vi "UI Initialize.vi"(8 "error in (no error)":errorcluster, 11 "UI ActorTop in":refnum<class "ButtonUI.lvclass">) -> (0 "error out":errorcluster, 3 "UI ActorTop out":refnum<class "ButtonUI.lvclass">)   [LabVIEW 2021, in "ButtonUI.lvclass"]
doc: "UI: Initialize\n2015-03-18 16:27:22\n蒋松\njiangsong@outlook.com"
uses:
  ButtonUI.lvclass
  ButtonUI.lvclass/ButtonUI.ctl
  <userlib>/John_Lib/AbstractActorTemplate/AbstractActorTemplate/UIActorTop.lvclass
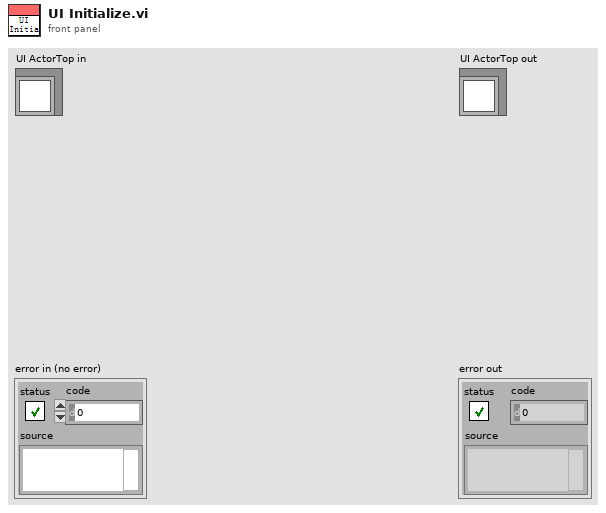
[diagram p1: front panel]
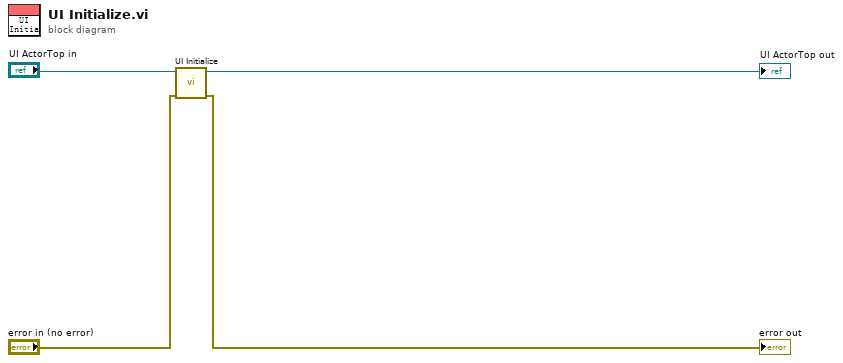
[diagram p0: block diagram]
diagram:
  n1 = call-parent "UI Initialize.vi"("error in (no error)"="error in (no error)", "UI ActorTop in"="UI ActorTop in") -> ("error out"=→"error out":errorcluster, "UI ActorTop out"=→"UI ActorTop out":refnum<class "ButtonUI.lvclass">)  [unwired: 8 in]
